vi "CRYSet Prompt Front Panel.vi"(11 "Vi Ref":refnum<vi>) -> ()   [LabVIEW 2013]
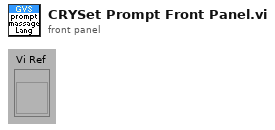
[diagram p1: front panel]
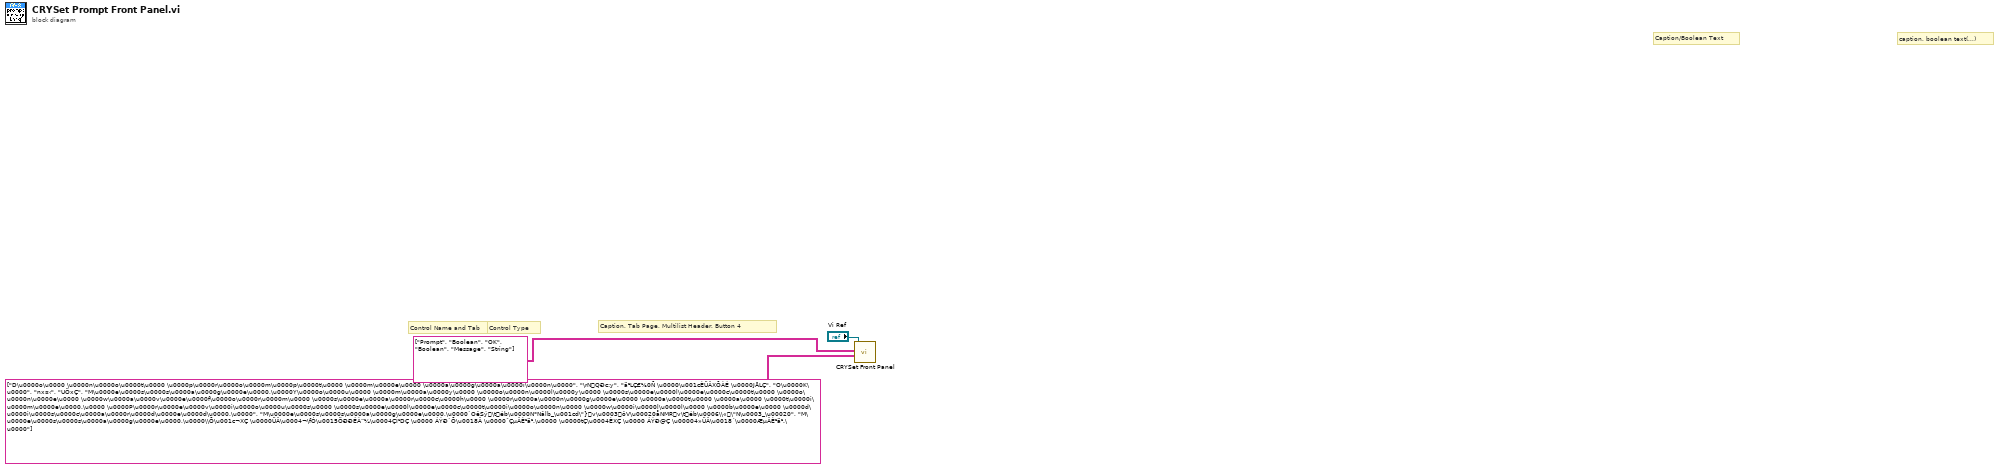
[diagram p0: block diagram]
diagram:
  # "Caption, Tab Page, Multilist Header, Button 4"
  # "Control Type"
  # "Control Name and Tab"
  # "caption, boolean text(,,,)"
  # "Caption/Boolean Text"
  n1 = call "CRYSet Front Panel.vi"("Caption(Boolean Text)"=string[][] [["D\u0000o\u0000 \u0000n\u0000o\u0000t\u0000 \u0000p\u0000r\u0000o\u0000m\u0000p\u0000t\u0000 \u0000m\u0000e\u0000 \u0000a\u0000g\u0000a\u0000i\u0000n\u0000", "\rNQÐc:y", "ä²LÇ€½0Ñ \u0000\u001cÈÜÂXÕÀÉ \u0000JÅLÇ"], ["O\u0000K\u0000", "nx¤‹", "UÖxÇ"], ["M\u0000e\u0000s\u0000s\u0000a\u0000g\u0000e\u0000,\u0000Y\u0000o\u0000u\u0000 \u0000m\u0000a\u0000y\u0000 \u0000o\u0000n\u0000l\u0000y\u0000 \u0000s\u0000e\u0000l\u0000e\u0000c\u0000t\u0000 \u0000o\u0000n\u0000e\u0000 \u0000w\u0000a\u0000v\u0000e\u0000f\u0000o\u0000r\u0000m\u0000 \u0000s\u0000e\u0000a\u0000r\u0000c\u0000h\u0000 \u0000r\u0000a\u0000n\u0000g\u0000e\u0000 \u0000a\u0000t\u0000 \u0000a\u0000 \u0000t\u0000i\u0000m\u0000e\u0000.\u0000 \u0000P\u0000r\u0000e\u0000v\u0000i\u0000o\u0000u\u0000s\u0000 \u0000s\u0000e\u0000l\u0000e\u0000c\u0000t\u0000i\u0000o\u0000n\u0000 \u0000w\u0000i\u0000l\u0000l\u0000 \u0000b\u0000e\u0000 \u0000d\u0000i\u0000s\u0000c\u0000a\u0000r\u0000d\u0000e\u0000d\u0000.\u0000", "M\u0000e\u0000s\u0000s\u0000a\u0000g\u0000e\u0000,\u0000`OêSý\téb\u0000N*Nâlb_\u001cd\"}v\u0003ôV\u00020åNMRv\téb\u0006\\«\"N\u0003_\u00020", "M\u0000e\u0000s\u0000s\u0000a\u0000g\u0000e\u0000,\u0000\\Õ\u001c¬XÇ \u0000ÜÂ\u0004¬\fÓ\u0015ÖÐÐÉÀ”¼\u0004ÇÌ¹DÇ \u0000 ÁÝÐ`Õ\u0018Â \u0000ˆÇµÂÈ²ä².\u0000 \u0000tÇ\u0004ÈXÇ \u0000 ÁÝÐ@Ç \u00004»ÜÂ\u0018´\u0000ÆµÂÈ²ä².\u0000"]], "Control ID and Type(Label Name, Type)"=string[][] [["Prompt", "Boolean"], ["OK", "Boolean"], ["Message", "String"]], "Vi Ref"="Vi Ref") -> ()  [unwired: 9 in]
